vi "Amplitude and Levels (obs).vi"   [LabVIEW 2020, in "NI_MAPro.lvlib"]
uses:
  NI_MAPro.lvlib
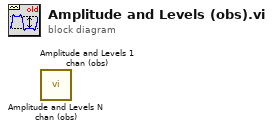
[diagram p0: block diagram]
diagram:
  n1 = call "Amplitude and Levels N chan (obs).vi"() -> ()  [unwired: 8 in, 4 out]
  n2 = call "Amplitude and Levels 1 chan (obs).vi"() -> ()  [unwired: 8 in, 4 out]
